vi "Get Heartbeat Checker Execution State.vi"(8 "error in":errorcluster, 11 "CANopen Master in":refnum<class "CANopen Master.lvclass">) -> (0 "error out":errorcluster, 2 "Execution:State":T1(ring), 3 "CANopen Master out":refnum<class "CANopen Master.lvclass">)   [LabVIEW 2024, in "CANopen Master.lvlib" / "CANopen Master.lvclass"]
uses:
  CANopen Master.lvclass
  CANopen Master.lvclass/CANopen Master.ctl
  Example/Network Management/Network Mangement.lvclass
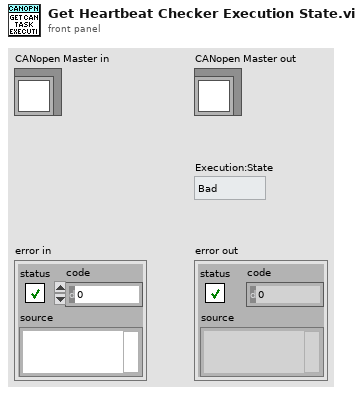
[diagram p1: front panel]
types:
  T1 = enum32{"Bad", "Idle", "Run top level", "Running"}
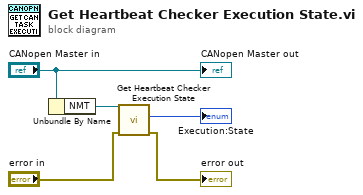
[diagram p0: block diagram]
diagram:
  n1 = Unbundle By Name("CANopen Master in") -> ("NMT"=w4:refnum<class "Network Mangement.lvclass">)
  n2 = call "Get Heartbeat Checker Execution State.vi"("Error In"="error in", "reference in"=w4) -> ("Error Out"=→"error out":errorcluster, "Exec.State"=→"Execution:State":T1)  [unwired: 7 in, 1 out]
  "CANopen Master out" <- "CANopen Master in"
